vi "MJSort_Fun.vi"(10 "Old Files":T1[](array[typedef])) -> ()   [LabVIEW 2022 SP3]
uses:
  Curtin1_Label.ctl
panel:
  out "Files":picture
  out "X":i32
  out "FRF":cluster{"x0":dbl, "df":dbl, dbl[]}[](graph)
  # "Welcome to MJs sorting\n\nThis lets you sort by any vertical position in the plot - just move the cursor.  Note the order changes below."
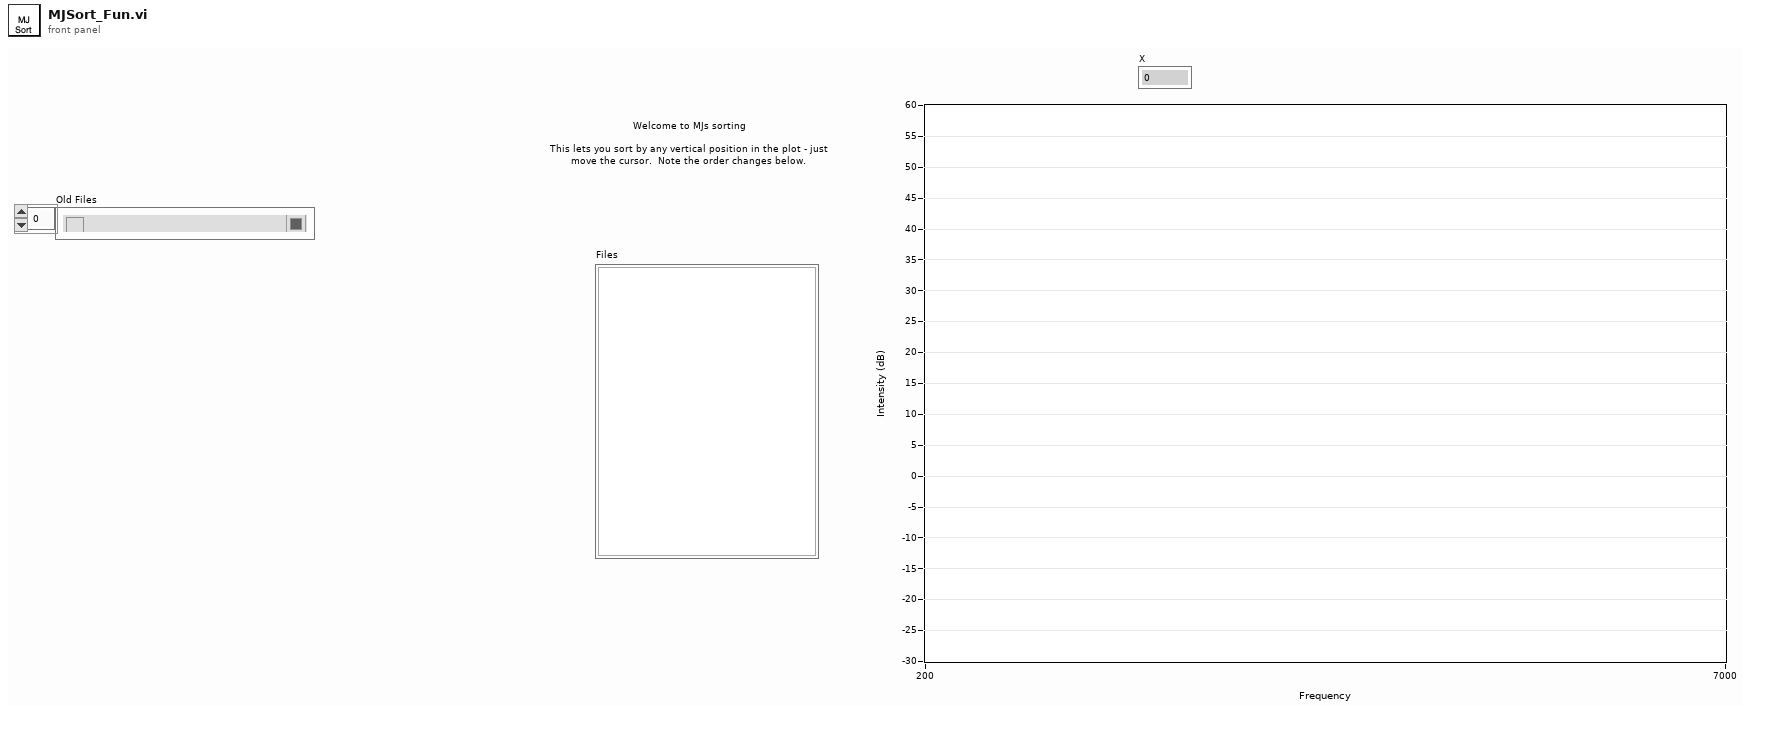
[diagram p1: front panel]
types:
  T1 = typedef "Curtin1_Label.ctl" = cluster{"Show?":bool, "Name":string, "Color":u32, "Path":path, "Show Notes":bool}
  T2 = cluster{"left":i16, "top":i16, "right":i16, "bottom":i16}
  T3 = cluster{"Start freq":dbl, "Hz resolution":dbl, cdb[]}
  T4 = cluster{"count (1)":dbl, "Name":string, i32, "Color":u32}
  T5 = cluster{"count (1)":dbl, "Name":string, i32, "Color":u32}[]
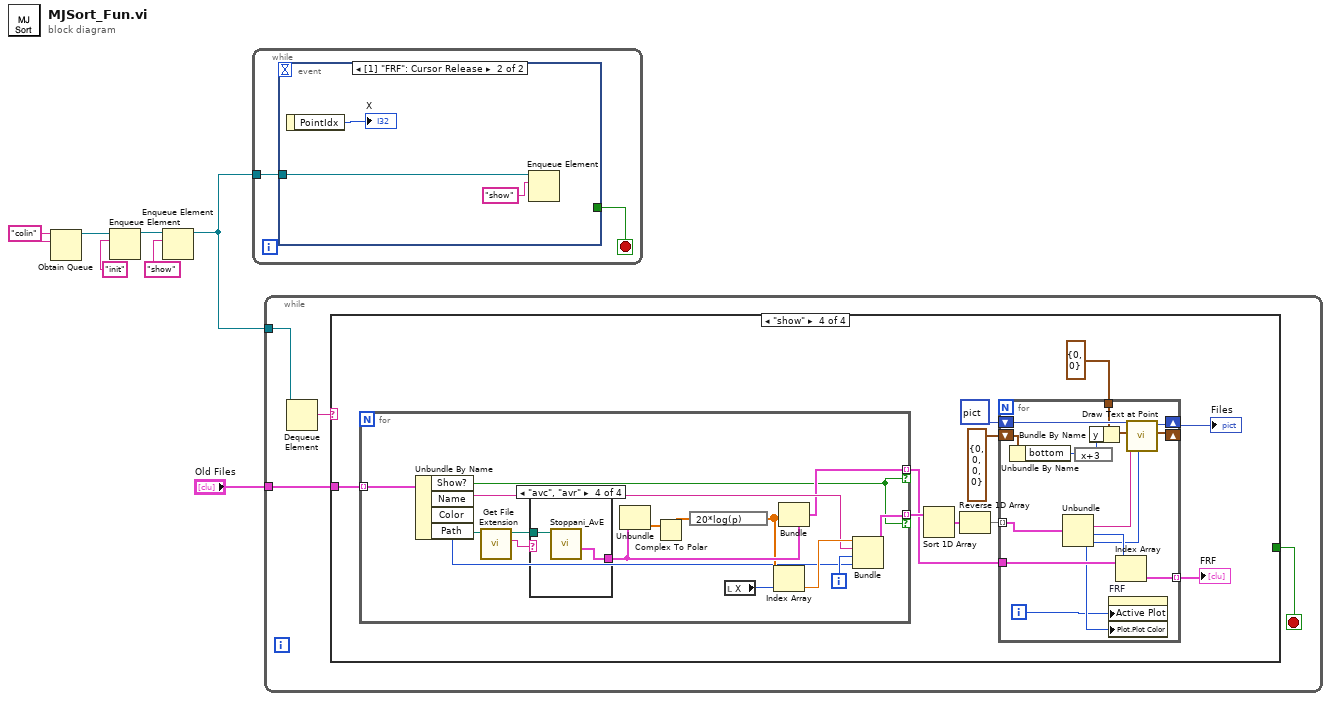
[diagram p0: block diagram]
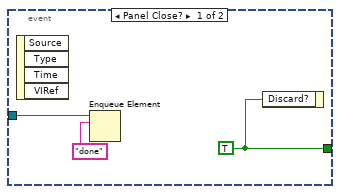
[diagram p2: hidden frame]
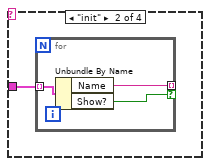
[diagram p4: hidden frame]
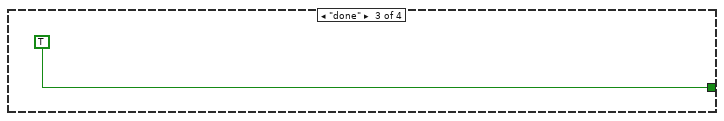
[diagram p5: hidden frame]
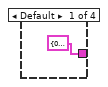
[diagram p6: hidden frame]
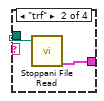
[diagram p7: hidden frame]
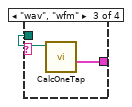
[diagram p8: hidden frame]
diagram:
  w7 = "colin" ("name (unnamed)")
  n1 = Obtain Queue(name (unnamed)=w7, element data type=w7) -> (queue out=w2:refnum<queue>)  [unwired: 3 in, 2 out]
  n2 = Enqueue Element(queue=w2, element="init") -> (queue out=w1:refnum<queue>)  [unwired: 2 in, 2 out]
  n3 = Enqueue Element(queue=w1, element="show") -> (queue out=w5:refnum<queue>)  [unwired: 2 in, 2 out]
  n4 = while {
    tunnel: w5 -> [w8]
    stop <- w9 stop-if-true
    n5 = event shown="[1] \"FRF\": Cursor Release" {
      selector: _ -> [_ _]
      dyn-events: _ -> [_ _]
      timeout: _ -> [_ _]
      tunnel: [w10 _] -> w9
      tunnel: w8 -> [w11 w15]
      event Panel Close? {
        w10 = TRUE
        n6 = event-data() -> ()  [unwired: 1 in, 4 out]
        n7 = Enqueue Element(queue=w11, element="done") -> ()  [unwired: 2 in, 3 out]
        n8 = event-data("Discard?"=w10) -> ()  [unwired: 1 in, 1 out]
      }
      event "FRF": Cursor Release {
        n9 = event-data() -> ("PointIdx"=→"X":i32)  [unwired: 1 in]
        n10 = Enqueue Element(queue=w15, element="show") -> ()  [unwired: 2 in, 3 out]
      }
    }
  }
  n11 = while {
    tunnel: w5 -> [w19]
    tunnel: "Old Files" -> [w16]
    stop <- w17 stop-if-true
    n12 = Dequeue Element(queue=w19) -> (element=w18:string)  [unwired: 2 in, 3 out]
    n13 = case shown="\"show\"" w18 {
      tunnel: [_ _ TRUE _] -> w17
      tunnel: w16 -> [_ w20 _ w34]
      frame Default {
      }
      frame "init" {
        n14 = for {
          tunnel: w20 -> [w23] mode=indexing
          tunnel: [w22] -> _ mode=indexing if=w21
          n15 = Unbundle By Name(w23) -> ("Name"=w22:string, "Show?"=w21:bool)
        }
      }
      frame "done" {
      }
      frame "show" {
        n16 = for {
          tunnel: w34 -> [w59] mode=indexing
          tunnel: [w55] -> w33 mode=indexing if=w51
          tunnel: [w52] -> w31 mode=indexing if=w51
          i -> [w53]
          n17 = Unbundle By Name(w59) -> ("Show?"=w51:bool, "Name"=w54:string, "Color"=w50:u32, "Path"=w65:path)
          n18 = call <vilib>:"Get File Extension.vi"("file"=w65) -> ("lowercase file extension"=w63:string, "dup file"=w64:path)  [unwired: 6 in, 3 out]
          n19 = case shown="\"avc\", \"avr\"" w63 {
            tunnel: [T3 {"Start freq"=0.0, "Hz resolution"=0.0, []} ("Waveform Graph") w67 w69 w72] -> w61
            tunnel: w64 -> [_ w68 w70 w71]
            frame Default {
            }
            frame "trf" {
              n20 = call "Stoppani File Read.vi"("String in"=w68) -> ("Complex FRF"=w67:cluster{"t0":dbl, "dt":dbl, "Y":cdb[]})  [unwired: 2 in, 3 out]
            }
            frame "wav", "wfm" {
              n21 = call "CalcOneTap.vi"("wavform file"=w70) -> ("Complex FRF"=w69:cluster{dbl, "df":dbl, cdb[]})  [unwired: 7 in, 3 out]
            }
            frame "avc", "avr" {
              n22 = call "Stoppani_AvE.vi"("file (use dialog)"=w71) -> ("Complex FRF"=w72:cluster{"t0":dbl, "df":dbl, "Y":cdb[]})  [unwired: 7 in, 3 out]
            }
          }
          n23 = Unbundle(w61) -> ("Y"=w62:cdb[])  [unwired: 2 out]
          n24 = Complex To Polar(r * e^(i*theta)=w62) -> (r=w60:dbl[])  [unwired: 1 out]
          n25 = expression code="20*log(p)"(w60) -> (w57:dbl[])
          n26 = local read "X"() -> (w58:i32)
          n27 = Index Array(array=w57, index=w58) -> (element=w56:dbl)
          n28 = Bundle(cluster=w61, "Y"=w57) -> (w52:cluster{"t0":dbl, "df":dbl, "Y":cdb[]})  [unwired: 2 in]
          n29 = Bundle("count (1)"=w56, "Name"=w54, w53, "Color"=w50) -> (w55:T4)  [unwired: 1 in]
        }
        n30 = Sort 1D Array(array=w33) -> (sorted array=w32:T5)
        n31 = Reverse 1D Array(array=w32) -> (reversed array=w25:T5)
        n32 = for {
          tunnel: w25 -> [w49] mode=indexing
          tunnel: w31 -> [w48]
          tunnel: [w46] -> w30 mode=indexing
          shift-right: [w44] -> w28
          shift-left: picture data[5B] ("Files") -> [w45]
          tunnel: cluster{"x":i16, "y":i16} {"x"=0, "y"=0} ("origin") -> [w41]
          shift-right: [w38] -> _
          shift-left: T2 {"left"=0, "top"=0, "right"=0, "bottom"=0} ("text rect") -> [w37]
          i -> [w39]
          n33 = Unbundle By Name(w37) -> ("bottom"=w36:i16)
          n34 = Unbundle(w49) -> ("Name"=w43:string, w47:i32, "Color"=w42:u32)  [unwired: 1 out]
          n35 = expression code="x+3"(w36) -> (w35:i16)
          n36 = Bundle By Name(cluster=w41, "y"=w35) -> (w40:cluster{"x":i16, "y":i16})
          n37 = property on="FRF" class="WFGraph (strict)"("Active Plot"=w39, "Plot.Plot Color"=w42) -> ()  [unwired: 2 in, 2 out]
          n38 = Index Array(array=w48, index=w47) -> (element=w46:cluster{"t0":dbl, "df":dbl, "Y":cdb[]})
          n39 = call <vilib>:"Draw Text at Point.vi"("text color(black)"=w42, "text"=w43, "origin"=w40, "picture"=w45) -> ("text rect"=w38:T2, "new picture"=w44:picture)  [unwired: 6 in]
        }
        "FRF" <- w30
        "Files" <- w28
      }
    }
  }
